vi "Запись в файл (SubVI).vi"(8 "error in":errorcluster, 10 "Строка параметров мишеней для сохранения":string) -> (0 "error out":errorcluster, 3 "путь к файлу ref":refnum<file>, 5 "Путь к файлу":path)   [LabVIEW 2015]
doc: "Сохранение текущей конфигурации в файл Настройки.txt, расположенный в каталоге с исполняемым файлом"
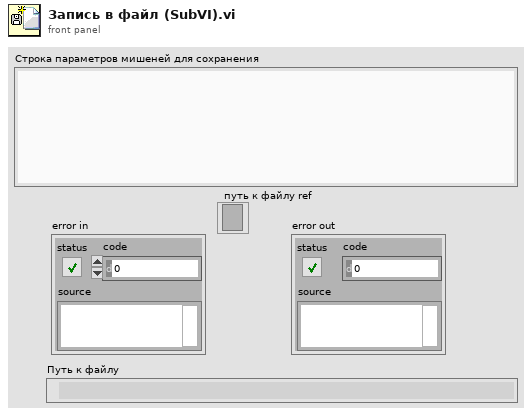
[diagram p1: front panel]
types:
  T1 = enum16{"open", "replace", "create", "open or create", "replace or create", "replace or create with confirmation"}
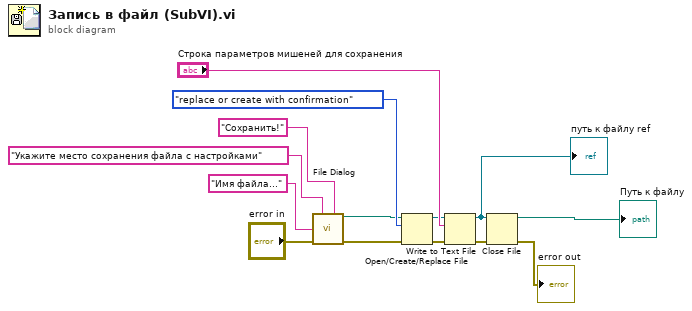
[diagram p0: block diagram]
diagram:
  n1 = call "File Dialog"("prompt"="Укажите место сохранения файла с настройками" ("string"), "button label"="Сохранить!" ("string"), "default name"="Имя файла..." ("string"), "error in"="error in") -> ("selected path"=w2:path, "error out"=w6:errorcluster)  [unwired: 8 in, 2 out]
  n2 = Open/Create/Replace File(file path (use dialog)=w2, error in=w6, operation (0:open)=T1."replace or create with confirmation") -> (refnum out=w11:refnum<file>, error out=w9:errorcluster)  [unwired: 4 out]
  n3 = Write to Text File(file (use dialog)=w11, text="Строка параметров мишеней для сохранения", error in=w9) -> (refnum out=w13:refnum<file>, error out=w12:errorcluster)  [unwired: 2 out]
  "путь к файлу ref" <- w13
  n4 = Close File(refnum=w13, error in=w12) -> (path=→"Путь к файлу":path, error out=→"error out":errorcluster)
